vi "Serial_read.vi"(7 "Read mode":enum16{"Read all", "Get latest value"}(ring)=enum."Get latest value", 8 "error in (no error)":errorcluster, 10 "Bytes at Port":u32, 11 "VISA Refnum in":refnum<visa-resource-name>) -> (0 "error out":errorcluster, 1 "dt":u32, 2 "read buffer":string, 3 "VISA resource name out":refnum<visa-resource-name>)   [LabVIEW 2017]
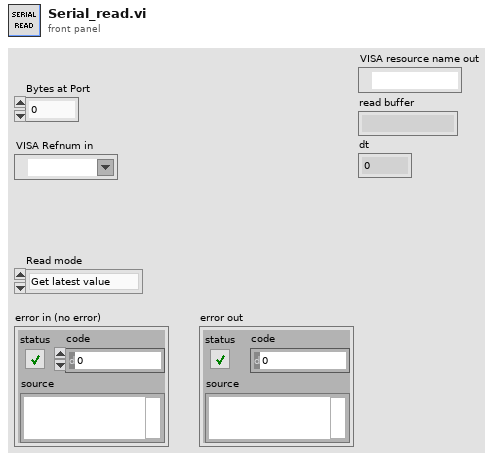
[diagram p1: front panel]
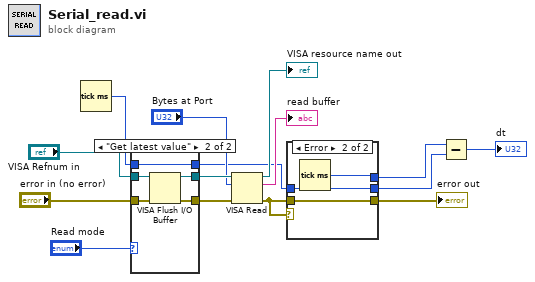
[diagram p0: block diagram]
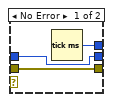
[diagram p2: hidden frame]
diagram:
  n1 = Tick Count (ms)() -> (millisecond timer value=w5:u32)
  n2 = case shown="\"Get latest value\"" "Read mode" {
    tunnel: "error in (no error)" -> [w18 w23]
    tunnel: [w18 w21] -> w15
    tunnel: [w17 w22] -> w14
    tunnel: "VISA Refnum in" -> [w17 w20]
    tunnel: w5 -> [w16 w19]
    tunnel: [w16 w19] -> w4
    frame "Read all", Default {
    }
    frame "Get latest value" {
      n3 = VISA Flush I/O Buffer(VISA resource name=w20, error in (no error)=w23) -> (VISA resource name out=w22:refnum<visa-resource-name>, error out=w21:errorcluster)  [unwired: 1 in]
    }
  }
  n4 = VISA Read(VISA resource name=w14, byte count="Bytes at Port", error in (no error)=w15) -> (VISA resource name out=→"VISA resource name out":refnum<visa-resource-name>, read buffer=→"read buffer":string, error out=w6:errorcluster)  [unwired: 1 out]
  n5 = case shown="Error" w6 {
    tunnel: w6 -> [w26 w27]
    tunnel: [w26 w27] -> w7
    tunnel: w4 -> [w25 w28]
    tunnel: [w25 w28] -> w3
    tunnel: [w24 w29] -> w2
    frame No Error {
      n6 = Tick Count (ms)() -> (millisecond timer value=w24:u32)
    }
    frame Error {
      n7 = Tick Count (ms)() -> (millisecond timer value=w29:u32)
    }
  }
  "error out" <- w7
  n8 = Subtract(x=w2, y=w3) -> (x-y=→"dt":u32)
